vi "Elapsed time.vi"(7 "Name":string="default", 8 "err in":errorcluster, 9 "Sec to wait (10)":dbl=10.0, 10 "Mode":enum16{"Get", "Reset"}(ring)) -> (0 "err out":errorcluster, 1 "Elapsed?":bool, 2 "Elapsed sec":dbl)   [LabVIEW 2019, in "Sending_larger_data.lvlib"]
uses:
  Sending_larger_data.lvlib
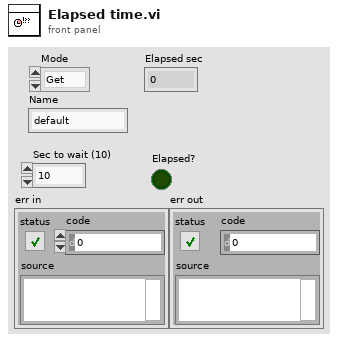
[diagram p1: front panel]
types:
  T1 = cluster{"seconds since 1Jan1904":timestamp, "name":string}
  T2 = cluster{"seconds since 1Jan1904":timestamp, "name":string}[]
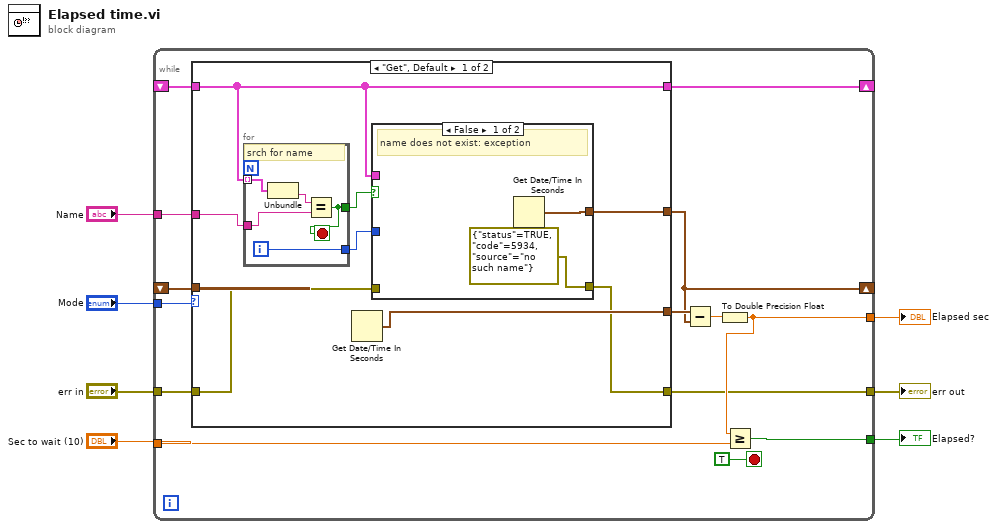
[diagram p0: block diagram]
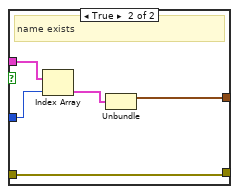
[diagram p2: hidden frame]
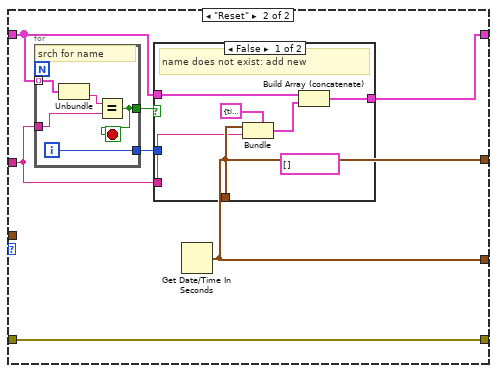
[diagram p3: hidden frame]
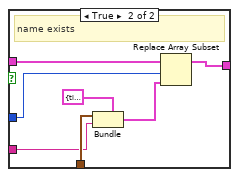
[diagram p4: hidden frame]
diagram:
  n1 = while {
    tunnel: "Mode" -> [w21]
    shift-right: [w18] -> _
    shift-left: _ -> [w20]
    tunnel: [w15] -> w7
    tunnel: "Sec to wait (10)" -> [w14]
    tunnel: [w13] -> w4
    tunnel: "Name" -> [w12]
    shift-right: [w11] -> _
    shift-left: _ -> [w10]
    tunnel: "err in" -> [w9]
    tunnel: [w8] -> w1
    stop <- TRUE stop-if-true
    n2 = case shown="\"Get\", Default" w21 {
      tunnel: [w24 w46] -> w18
      tunnel: w20 -> [_ _]
      tunnel: [w29 w46] -> w19
      tunnel: w12 -> [w28 w45]
      tunnel: [w25 w43] -> w11
      tunnel: w10 -> [w25 w44]
      tunnel: w9 -> [w23 w42]
      tunnel: [w22 w42] -> w8
      frame "Get", Default {
        n3 = for {
          tunnel: w25 -> [w41] mode=indexing
          tunnel: w28 -> [w39]
          tunnel: [w38] -> w27
          tunnel: [w37] -> w26
          i -> [w37]
          stop <- w38 stop-if-true
          # "srch for name"
          n4 = Unbundle(w41) -> ("name"=w40:string)  [unwired: 1 out]
          n5 = Equal?(x=w40, y=w39) -> (x = y?=w38:bool)
        }
        n6 = Get Date/Time In Seconds() -> (seconds since 1Jan1904=w29:timestamp)
        n7 = case shown="False" w27 {
          tunnel: w26 -> [_ w35]
          tunnel: w25 -> [_ w36]
          tunnel: [w31 w33] -> w24
          tunnel: w23 -> [_ w32]
          tunnel: [errorcluster {"status"=TRUE, "code"=5934, "source"="no such name"} ("error constant") w32] -> w22
          frame False {
            # "name does not exist: exception"
            n8 = Get Date/Time In Seconds() -> (seconds since 1Jan1904=w31:timestamp)
          }
          frame True {
            # "name exists"
            n9 = Index Array(array=w36, index=w35) -> (element=w34:T1)
            n10 = Unbundle(w34) -> ("seconds since 1Jan1904"=w33:timestamp)  [unwired: 1 out]
          }
        }
      }
      frame "Reset" {
        n11 = for {
          tunnel: w44 -> [w66] mode=indexing
          tunnel: w45 -> [w64]
          tunnel: [w63] -> w48
          tunnel: [w62] -> w47
          i -> [w62]
          stop <- w63 stop-if-true
          # "srch for name"
          n12 = Unbundle(w66) -> ("name"=w65:string)  [unwired: 1 out]
          n13 = Equal?(x=w65, y=w64) -> (x = y?=w63:bool)
        }
        n14 = Get Date/Time In Seconds() -> (seconds since 1Jan1904=w46:timestamp)
        n15 = case shown="False" w48 {
          tunnel: w47 -> [_ w57]
          tunnel: w46 -> [w53 w60]
          tunnel: w45 -> [w52 w59]
          tunnel: [w49 w56] -> w43
          tunnel: w44 -> [w51 w58]
          frame False {
            (unwired) T2 []
            # "name does not exist: add new"
            n16 = Bundle(cluster=T1 {"seconds since 1Jan1904"=timestamp(0 s since 1904-01-01), "name"=""}, "seconds since 1Jan1904"=w53, "name"=w52) -> (w50:T1)
            n17 = Build Array (concatenate)(w51, w50) -> (w49:T2)
          }
          frame True {
            # "name exists"
            n18 = Bundle(cluster=T1 {"seconds since 1Jan1904"=timestamp(0 s since 1904-01-01), "name"=""}, "seconds since 1Jan1904"=w60, "name"=w59) -> (w55:T1)
            n19 = Replace Array Subset(array=w58, new element=w55, index=w57) -> (w56:T2)
          }
        }
      }
    }
    n20 = Subtract(x=w19, y=w18) -> (x-y=w17:dbl)
    n21 = To Double Precision Float(number=w17) -> (double precision float=w15:dbl)
    n22 = Greater Or Equal?(x=w15, y=w14) -> (x >= y?=w13:bool)
  }
  "Elapsed sec" <- w7
  "Elapsed?" <- w4
  "err out" <- w1
